vi "Read Caption.vi"(9 "Control in":refnum<class "Control.lvclass">) -> (3 "Control out":refnum<class "Control.lvclass">, 4 "Caption":refnum<class "Text.lvclass">)   [LabVIEW 2014, in "Control.lvclass"]
uses:
  Control.lvclass
  Text/Text.lvclass
  Control.lvclass/Control.ctl
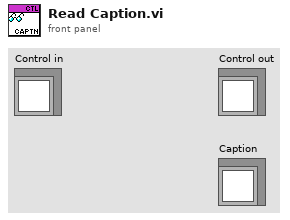
[diagram p1: front panel]
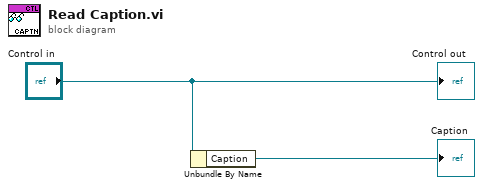
[diagram p0: block diagram]
diagram:
  n1 = Unbundle By Name("Control in") -> ("Caption"=→"Caption":refnum<class "Text.lvclass">)
  "Control out" <- "Control in"
